vi "Intake_motor_power.vi"(4 "Open_Man":bool, 5 "Carry_Auto":bool, 6 "Open_Step":bool, 7 "Open_Station":bool, 8 "Open_Score":bool, 9 "Station_Infeed_cmd":dbl min=-1.0 max=1.0 step=1.0, 10 "Infeed_Man_cmd":dbl, 11 "Floor_Infeed_cmd":dbl min=-1.0 max=1.0 step=1.0) -> (2 "Infeed_Pneu":bool, 3 "Intake_Power":dbl)   [LabVIEW 2014]
uses:
  General_VI/Global Var.vi
panel:
  in  "Auto_Infeed_Override":bool
  in  "Power Multiplier":dbl=1.0
  # "Intake Motor Control - Manual control will override automatic intake controls.\nValues for auto control are strictly integers and range from [-1,1].\nManual control values are all numbers from [-1,1]."
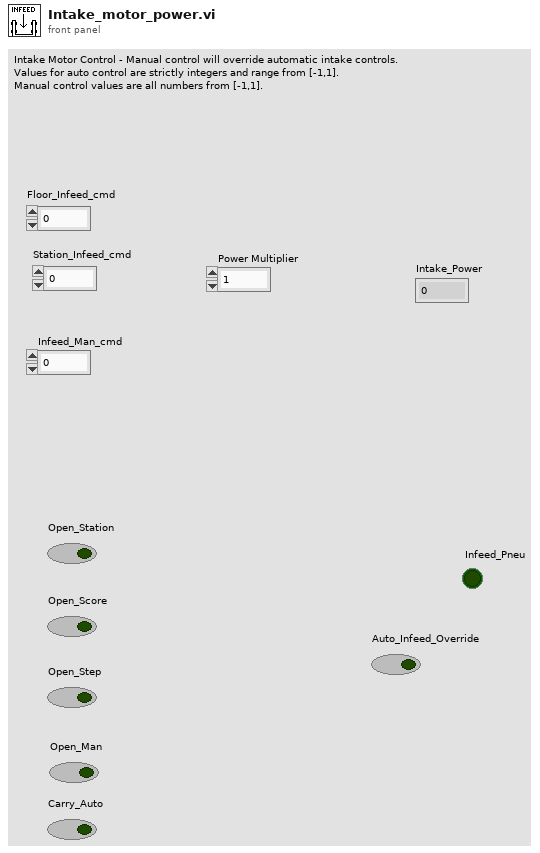
[diagram p1: front panel]
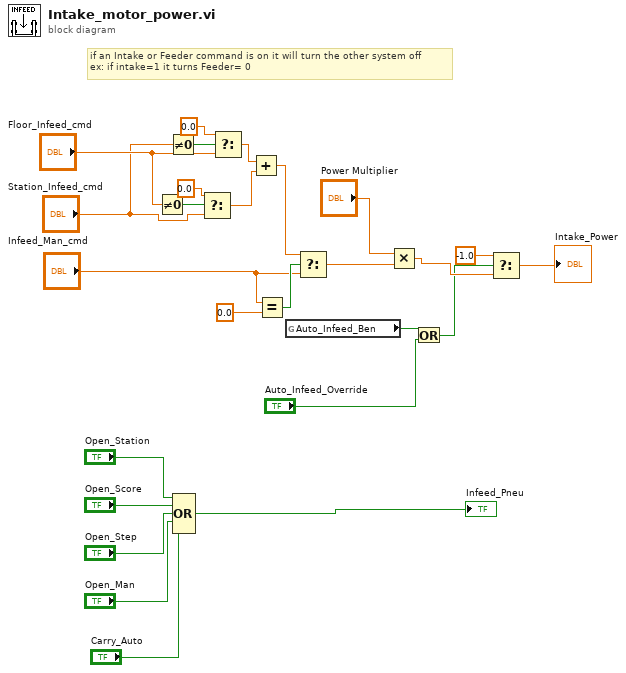
[diagram p0: block diagram]
diagram:
  # "if an Intake or Feeder command is on it will turn the other system off\nex: if intake=1 it turns Feeder= 0"
  n1 = Not Equal To 0?(x="Floor_Infeed_cmd") -> (x != 0?=w20:bool)
  n2 = Not Equal To 0?(x="Station_Infeed_cmd") -> (x != 0?=w17:bool)
  n3 = Compound Arithmetic op=OR("Open_Station", "Open_Score", "Open_Step", "Open_Man", "Carry_Auto") -> (→"Infeed_Pneu":bool)
  n4 = Select(t=0.0, s=w20, f="Station_Infeed_cmd") -> (s? t:f=w19:dbl)
  n5 = Select(t=0.0, s=w17, f="Floor_Infeed_cmd") -> (s? t:f=w13:dbl)
  n6 = Add(x=w13, y=w19) -> (x+y=w21:dbl)
  n7 = Equal?(x="Infeed_Man_cmd", y=0.0) -> (x = y?=w24:bool)
  n8 = global read "Global Var.vi" "Auto_Infeed_Ben"() -> (w3:bool)
  n9 = Select(t=w21, s=w24, f="Infeed_Man_cmd") -> (s? t:f=w25:dbl)
  n10 = Multiply(x="Power Multiplier", y=w25) -> (x*y=w6:dbl)
  n11 = Or(x=w3, y="Auto_Infeed_Override") -> (x .or. y?=w1:bool)
  n12 = Select(t=-1.0, s=w1, f=w6) -> (s? t:f=→"Intake_Power":dbl)
